vi "ExpVar AddNewExpVar.vi"(7 "VarType":T1(ring), 8 "error in (no error)":errorcluster, 9 "Var":variant, 10 "String label":string, 11 "ExpVar in":refnum<class "ExpVar.lvclass">) -> (0 "error out":errorcluster, 3 "NewExpVar out":refnum<class "ExpVar.lvclass">)   [LabVIEW 2018, in "ExpVar.lvclass"]
uses:
  ExpVar.lvclass
  ExpVar.lvclass/ExpVar.ctl
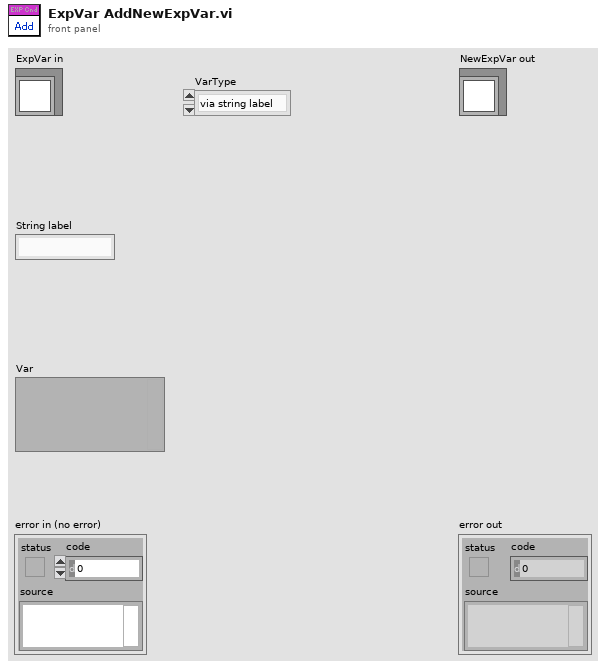
[diagram p1: front panel]
types:
  T1 = enum16{"via string label", "Laser", "Pressure", "TMP", "Script", "Signal Remarks", "ExtAO", "ExtDO", "ExtDI", "D999"}
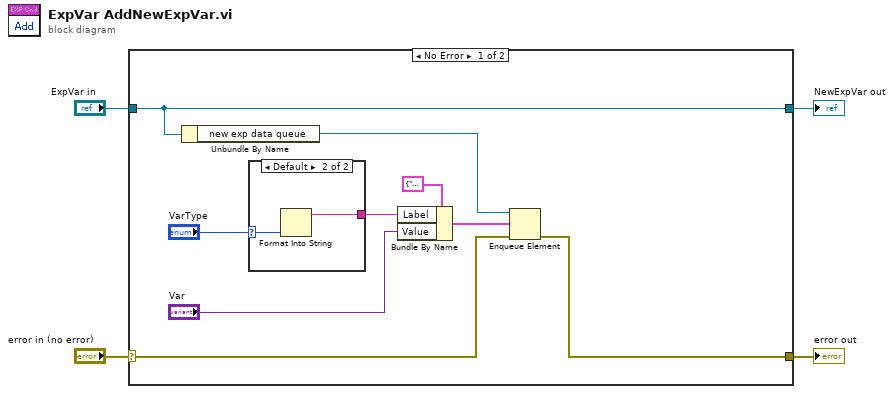
[diagram p0: block diagram]
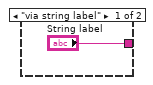
[diagram p2: hidden frame]
diagram:
  n1 = case shown="No Error" "error in (no error)" {
    selector: "error in (no error)" -> [w8 w18]
    tunnel: [w5 w18] -> w3
    tunnel: [w13 w17] -> w1
    tunnel: "ExpVar in" -> [w13 w17]
    frame No Error {
      n2 = Unbundle By Name(w13) -> ("new exp data queue"=w12:refnum<queue>)
      n3 = case shown="Default" "VarType" {
        selector: "VarType" -> [_ w15]
        tunnel: ["String label" w16] -> w10
        frame "via string label" {
        }
        frame Default {
          n4 = Format Into String(w15) -> (resulting string=w16:string)  [unwired: 3 in, 1 out]
        }
      }
      n5 = Bundle By Name(cluster=cluster{"Label":string, "Value":variant} {"Label"="", "Value"=variant} ("element"), "Label"=w10, "Value"="Var") -> (w9:cluster{"Label":string, "Value":variant})
      n6 = Enqueue Element(queue=w12, element=w9, error in (no error)=w8) -> (error out=w5:errorcluster)  [unwired: 1 in, 2 out]
    }
    frame Error {
    }
  }
  "error out" <- w3
  "NewExpVar out" <- w1
